vi "Get Waypoint Queue String.vi"(11 "Aircraft ID":u8) -> (3 "Aircraft Q Name":string)   [LabVIEW 2014]
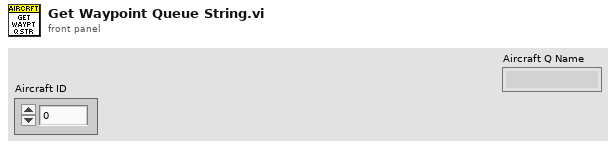
[diagram p1: front panel]
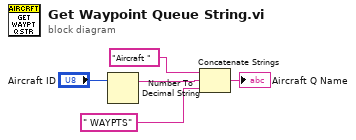
[diagram p0: block diagram]
diagram:
  n1 = Number To Decimal String(number="Aircraft ID") -> (decimal integer string=w3:string)  [unwired: 1 in]
  n2 = Concatenate Strings("Aircraft ", w3, " WAYPTS" ("string")) -> (→"Aircraft Q Name":string)
